vi "computeNamespace.vi"(7 "Build Namespace (F)":bool, 8 "error in (no error)":errorcluster, 10 "Name":string, 11 "Test Runner in":refnum<class "Test Runner.lvclass">) -> (0 "error out":errorcluster, 2 "Namespace":string, 3 "Test Runner out":refnum<class "Test Runner.lvclass">)   [LabVIEW 2013, in "Caraya.lvlib" / "Test Runner.lvclass"]
uses:
  Test Runner.lvclass
  <vilib>/regexp/Match Regular Expression.xnode
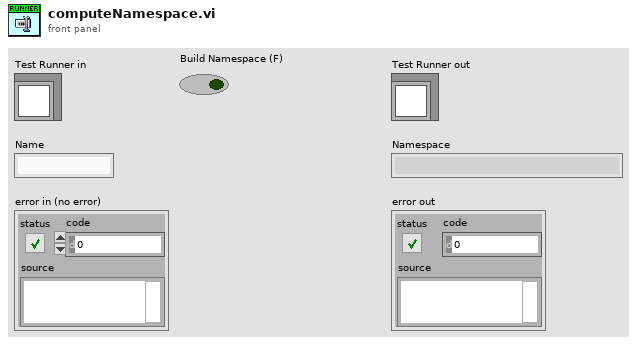
[diagram p1: front panel]
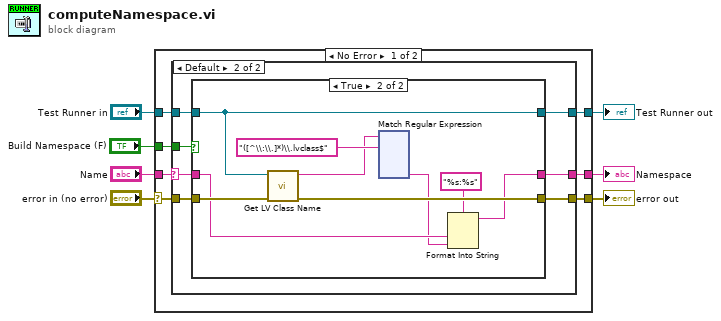
[diagram p0: block diagram]
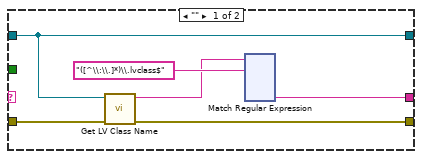
[diagram p2: hidden frame]
diagram:
  n1 = case shown="No Error" "error in (no error)" {
    selector: "error in (no error)" -> [w8 w273]
    tunnel: [w14 w273] -> w7
    tunnel: [w13 _] -> w6
    tunnel: [w12 w272] -> w5
    tunnel: "Test Runner in" -> [w11 w272]
    tunnel: "Name" -> [w10 _]
    tunnel: "Build Namespace (F)" -> [w9 _]
    frame No Error {
      n2 = case shown="Default" w10 {
        selector: w10 -> [_ w138]
        tunnel: [w15 w140] -> w13
        tunnel: w11 -> [w18 w141]
        tunnel: [w18 w137] -> w12
        tunnel: w8 -> [w20 w143]
        tunnel: [w19 w142] -> w14
        tunnel: w9 -> [_ w139]
        frame "" {
          n3 = call <vilib>:"Get LV Class Name.vi"("error in (no error)"=w20, "object"=w18) -> ("error out"=w19:errorcluster, "class name"=w16:string)  [unwired: 8 in]
          n4 = xnode "Match Regular Expression"("input string"=w16, "regular expression"="([^\\:\\.]*)\\.lvclass$") -> ("submatch 1"=w15:string)  [unwired: 4 in, 5 out]
        }
        frame Default {
          n5 = case shown="True" w139 {
            tunnel: w143 -> [w144 w155]
            tunnel: [w144 w154] -> w142
            tunnel: w141 -> [w145 w151]
            tunnel: [w146 w148] -> w140
            tunnel: w138 -> [w146 w150]
            tunnel: [w145 w151] -> w137
            frame False {
            }
            frame True {
              n6 = call <vilib>:"Get LV Class Name.vi"("error in (no error)"=w155, "object"=w151) -> ("error out"=w154:errorcluster, "class name"=w152:string)  [unwired: 8 in]
              n7 = xnode "Match Regular Expression"("input string"=w152, "regular expression"="([^\\:\\.]*)\\.lvclass$") -> ("submatch 1"=w149:string)  [unwired: 4 in, 5 out]
              n8 = Format Into String(format string="%s:%s", w150, w149) -> (resulting string=w148:string)  [unwired: 2 in, 1 out]
            }
          }
        }
      }
    }
    frame Error {
    }
  }
  "error out" <- w7
  "Namespace" <- w6
  "Test Runner out" <- w5
